vi "Set 1D Array Double Complex.vi"(5 "use temporary file?":bool, 7 "column vector?":bool, 8 "error in":errorcluster, 9 "value":cdb[](array[numeric]), 10 "variable name":string, 11 "GOLPI ref. in":T1={"pipe handle"={"lv_proc.dll file path"=path "", "process instance handle"=[]}, "fast read timeout [ms]"=500, "fast read settle time [ms]"=10, "fast read to multiple [ms]"=1, "max elements per input line"=100}) -> (0 "error out":errorcluster, 3 "GOLPI ref. out":T1={"pipe handle"={"lv_proc.dll file path"=path "", "process instance handle"=[]}, "fast read timeout [ms]"=500, "fast read settle time [ms]"=10, "fast read to multiple [ms]"=1, "max elements per input line"=100})   [LabVIEW 2013, in "GOLPI library.lvlib"]
uses:
  GOLPI library.lvlib
  Type Definitions/GOLPI reference Type Def.ctl
  LV Process.lvlibp/Pipe Handle.ctl
  LV Process.lvlibp
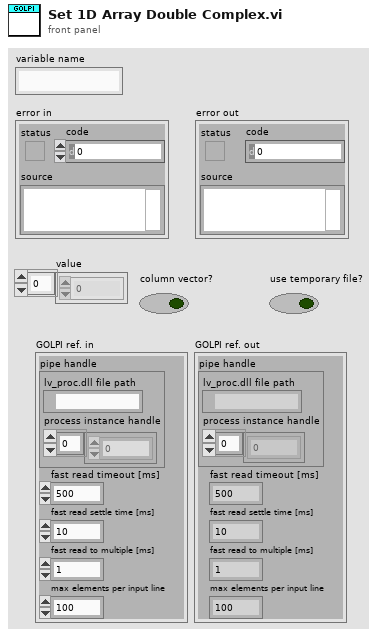
[diagram p1: front panel]
types:
  T1 = typedef "GOLPI library.lvlib/GOLPI reference Type Def.ctl" = cluster{"pipe handle":T2, "fast read timeout [ms]":u32, "fast read settle time [ms]":u32, "fast read to multiple [ms]":u32, "max elements per input line":u32}
  T2 = typedef "LV Process.lvlibp/Pipe Handle.ctl" = cluster{"lv_proc.dll file path":path, "process instance handle":u32[]}
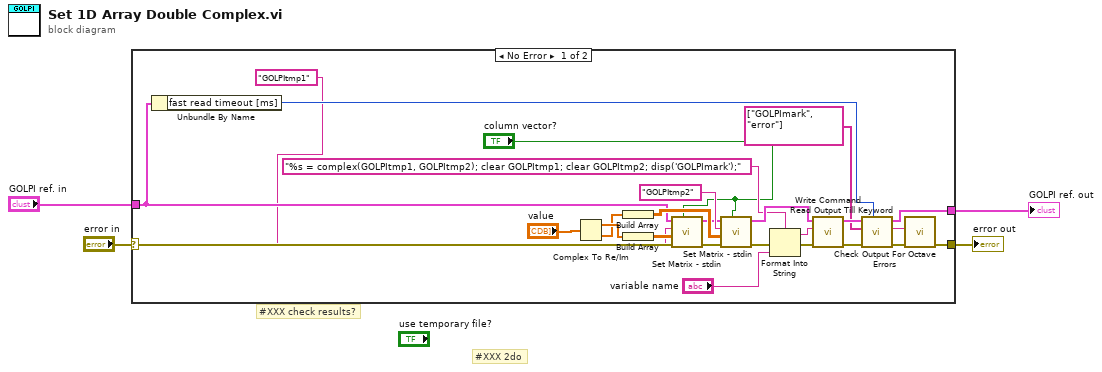
[diagram p0: block diagram]
diagram:
  # "#XXX 2do"
  # "#XXX check results?"
  n1 = case shown="No Error" "error in" {
    selector: "error in" -> [w30 w32]
    tunnel: [w10 w32] -> w4
    tunnel: "GOLPI ref. in" -> [w8 w31]
    tunnel: [w12 w31] -> w1
    frame No Error {
      n2 = Unbundle By Name(w8) -> ("fast read timeout [ms]"=w7:u32)
      n3 = Complex To Re/Im(x + iy="value") -> (x=w27:dbl[], y=w24:dbl[])
      n4 = Build Array(w24) -> (w25:dbl[][])
      n5 = Build Array(w27) -> (w29:dbl[][])
      n6 = call "Set Matrix - stdin.vi"("swap dimensions?"="column vector?", "error in"=w30, "value"=w29, "variable name"="GOLPItmp1", "GOLPI ref. in"=w8) -> ("error out"=w23:errorcluster, "GOLPI ref. out"=w22:T1)  [unwired: 5 in]
      n7 = call "Set Matrix - stdin.vi"("swap dimensions?"="column vector?", "error in"=w23, "value"=w25, "variable name"="GOLPItmp2", "GOLPI ref. in"=w22) -> ("error out"=w21:errorcluster, "GOLPI ref. out"=w20:T1)  [unwired: 5 in]
      n8 = Format Into String(format string="%s = complex(GOLPItmp1, GOLPItmp2); clear GOLPItmp1; clear GOLPItmp2; disp('GOLPImark');" ("command"), error in=w21, "variable name") -> (resulting string=w18:string, error out=w19:errorcluster)  [unwired: 1 in]
      n9 = call "Write Command.vi"("error in"=w19, "command"=w18, "GOLPI ref. in"=w20) -> ("error out"=w15:errorcluster, "GOLPI ref. out"=w14:T1)  [unwired: 7 in]
      n10 = call "Read Output Till Keyword.vi"("timeout [ms]"=w7, "error in"=w15, "keywords"=string[] ["GOLPImark", "error"], "GOLPI ref. in"=w14) -> ("error out"=w11:errorcluster, "read buffer"=w9:string, "GOLPI ref. out"=w12:T1)  [unwired: 4 in, 1 out]
      n11 = call "Check Output For Octave Errors.vi"("error in"=w11, "read buffer"=w9) -> ("error out"=w10:errorcluster)  [unwired: 9 in]
    }
    frame Error {
    }
  }
  "error out" <- w4
  "GOLPI ref. out" <- w1
